vi "config fpga resource.vi"(0 "fpga channel in":refnum<class "fpga channel.lvclass">, 1 "pairs in":T2[](array[typedef]), 2 "tagbus index":i32, 3 "bitfile ref in":refnum<k20>, 4 "hardware resource":T1, 5 "error in (no error)":errorcluster) -> (14 "fpga channel out":refnum<class "fpga channel.lvclass">, 15 "pairs out":T2[](array[typedef]), 19 "error out":errorcluster)   [LabVIEW 2015, in "fpga channel.lvclass"]
uses:
  fpga channel.lvclass
  execution/control index set.ctl
  <vilib>/NI/Tag Bus/tag/Data Type.ctl
  configuration/fpga resource supported data types.ctl
  <vilib>/NI/LVFPGA Adv Session Resources/ResourceInfo.ctl
  <vilib>/NI/Tag Bus/tag/tag descriptor.lvclass/tag descriptor.ctl
  fpga channel.lvclass/fpga channel.ctl
  <vilib>/NI/Tag Bus/tag/read data type.vi
  <vilib>/NI/Tag Bus/tag/read tag name.vi
  Read FXP type.vi
  execution/io runtime.lvclass
  <vilib>/NI/Configuration Framework/NISE_CEF_TreeControl.lvlib
  <vilib>/NI/Tag Bus/tag/tag descriptor.lvclass
  configuration/io configuration.lvclass
  <vilib>/NI/LVFPGA Adv Session Resources/LVFPGAAdvSessionResources.lvlib
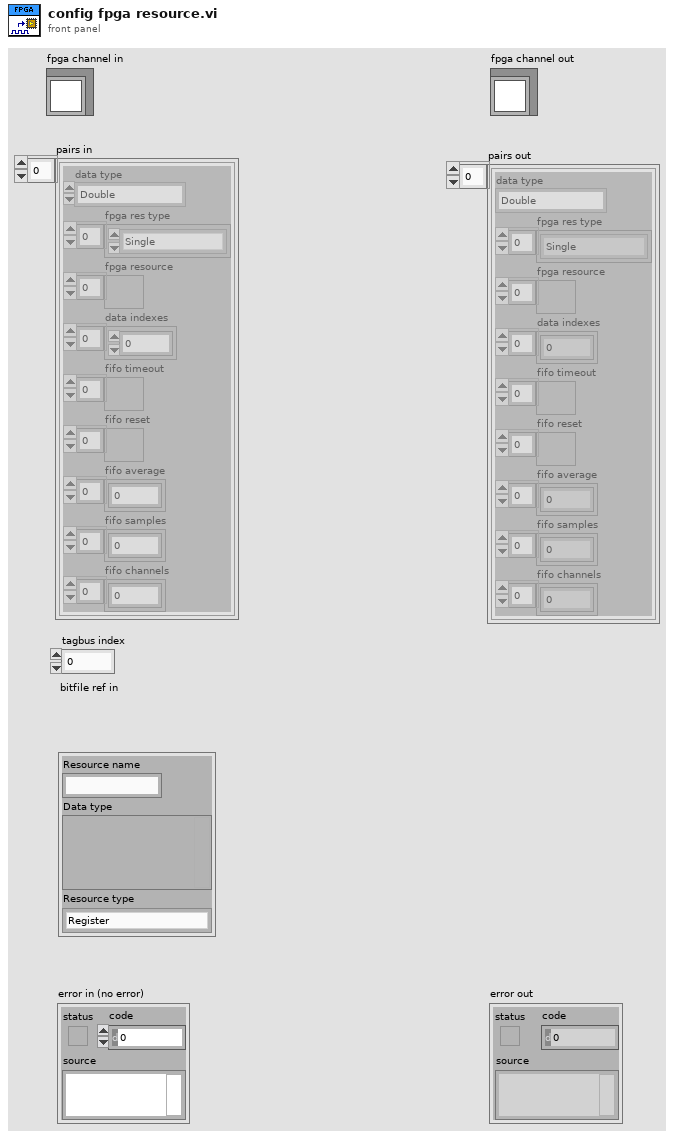
[diagram p1: front panel]
types:
  T1 = typedef "LVFPGAAdvSessionResources.lvlib/ResourceInfo.ctl" = cluster{"Resource name":string, "Data type":variant, "Resource type":enum16{"Register", "Host To Target FIFO", "Target To Host FIFO"}}
  T2 = typedef "io runtime.lvclass/control index set.ctl" = cluster{"data type":T3, "fpga res type":T4[], "fpga resource":refnum<k20>[], "data indexes":i32[], "fifo timeout":refnum<k20>[], "fifo reset":refnum<k20>[], "fifo average":i32[], "fifo samples":u32[], "fifo channels":u32[]}
  T3 = typedef "tag bus.lvlib/tag descriptor.lvclass/Data Type.ctl" = enum16{"Double", "Single", "I64", "I32", "I16", "I8", "U64", "U32", "U16", "U8", "Boolean", "String", "Array of Double", "Array of Single", "Array of I64", "Array of I32", "Array of I16", "Array of I8", "Array of U64", "Array of U32", "Array of U16", "Array of U8", "Array of Boolean", "Array of String"}
  T4 = typedef "io configuration.lvclass/fpga resource supported data types.ctl" = enum16{"Invalid Type", "Single", "I64", "I32", "I16", "I8", "U64", "U32", "U16", "U8", "Boolean", "FXP I,20,5", "FXP I,24,5", "FXP I,24,10", "Fifo 1023,I16"}
  T5 = typedef "LVFixedPointRepBitsTypeDef.ctl" = cluster{"Signed":bool, "Word Length":u32, "Integer Word Length":i32}
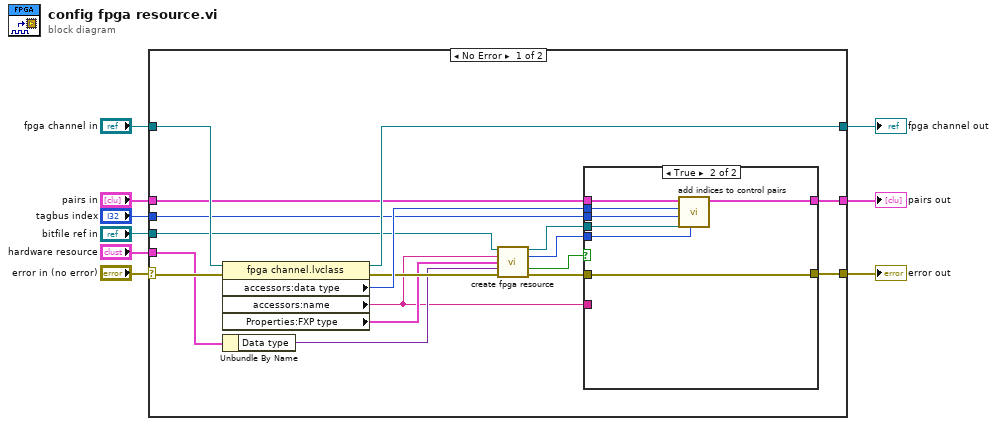
[diagram p0: block diagram]
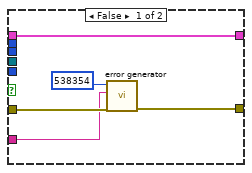
[diagram p2: hidden frame]
diagram:
  n1 = case shown="No Error" "error in (no error)" {
    selector: "error in (no error)" -> [w23 w42]
    tunnel: [w19 w42] -> w8
    tunnel: [w26 w41] -> w6
    tunnel: "fpga channel in" -> [w27 w41]
    tunnel: "pairs in" -> [w25 w40]
    tunnel: [w24 w40] -> w4
    tunnel: "bitfile ref in" -> [w16 _]
    tunnel: "tagbus index" -> [w21 _]
    tunnel: "hardware resource" -> [w20 _]
    frame No Error {
      n2 = property class="fpga channel.lvclass"(reference=w27, error in=w23) -> (reference out=w26:refnum<class "fpga channel.lvclass">, error out=w18:errorcluster, "accessors:data type"=w22:T3, "accessors:name"=w10:string, "Properties:FXP type"=w14:T5)
      n3 = Unbundle By Name(w20) -> ("Data type"=w13:variant)
      n4 = call "create fpga resource.vi"("Refnum in"=w16, "Resource name"=w10, "Channel FXP type"=w14, "Hardware Data type"=w13, "error in (no error)"=w18) -> ("Refnum out"=w15:refnum<k20>, "fpga res type"=w11:T4, "type supported"=w12:bool, "error out"=w17:errorcluster)  [unwired: 7 in]
      n5 = case shown="True" w12 {
        tunnel: [w31 w38] -> w24
        tunnel: w25 -> [w31 w39]
        tunnel: w21 -> [_ w36]
        tunnel: w22 -> [_ w37]
        tunnel: [w30 w35] -> w19
        tunnel: w17 -> [w29 w35]
        tunnel: w15 -> [_ w34]
        tunnel: w11 -> [_ w33]
        tunnel: w10 -> [w28 _]
        frame False {
          n6 = call <vilib>:"error generator.vi"("error in"=w29, "append error message"=w28, "error code (0)"=538354) -> ("error out"=w30:errorcluster)  [unwired: 6 in]
        }
        frame True {
          n7 = call "add indices to control pairs.vi"("fpga res type"=w33, "fpga resource"=w34, "data index"=w36, "data type"=w37, "pairs in"=w39) -> ("pairs out"=w38:T2[])  [unwired: 6 in]
        }
      }
    }
    frame Error {
    }
  }
  "error out" <- w8
  "fpga channel out" <- w6
  "pairs out" <- w4
